vi "Oversampler.vi"(9 "Samplerate":dbl format="%#_13g", 10 "Array in":dbl[](array[numeric]), 11 "Oversampling":i32=15) -> (3 "Array out":dbl[](array[numeric]))   [LabVIEW 2016]
panel:
  out "Waveform Graph 2":dbl[](graph)
  out "Waveform Graph":dbl[](graph)
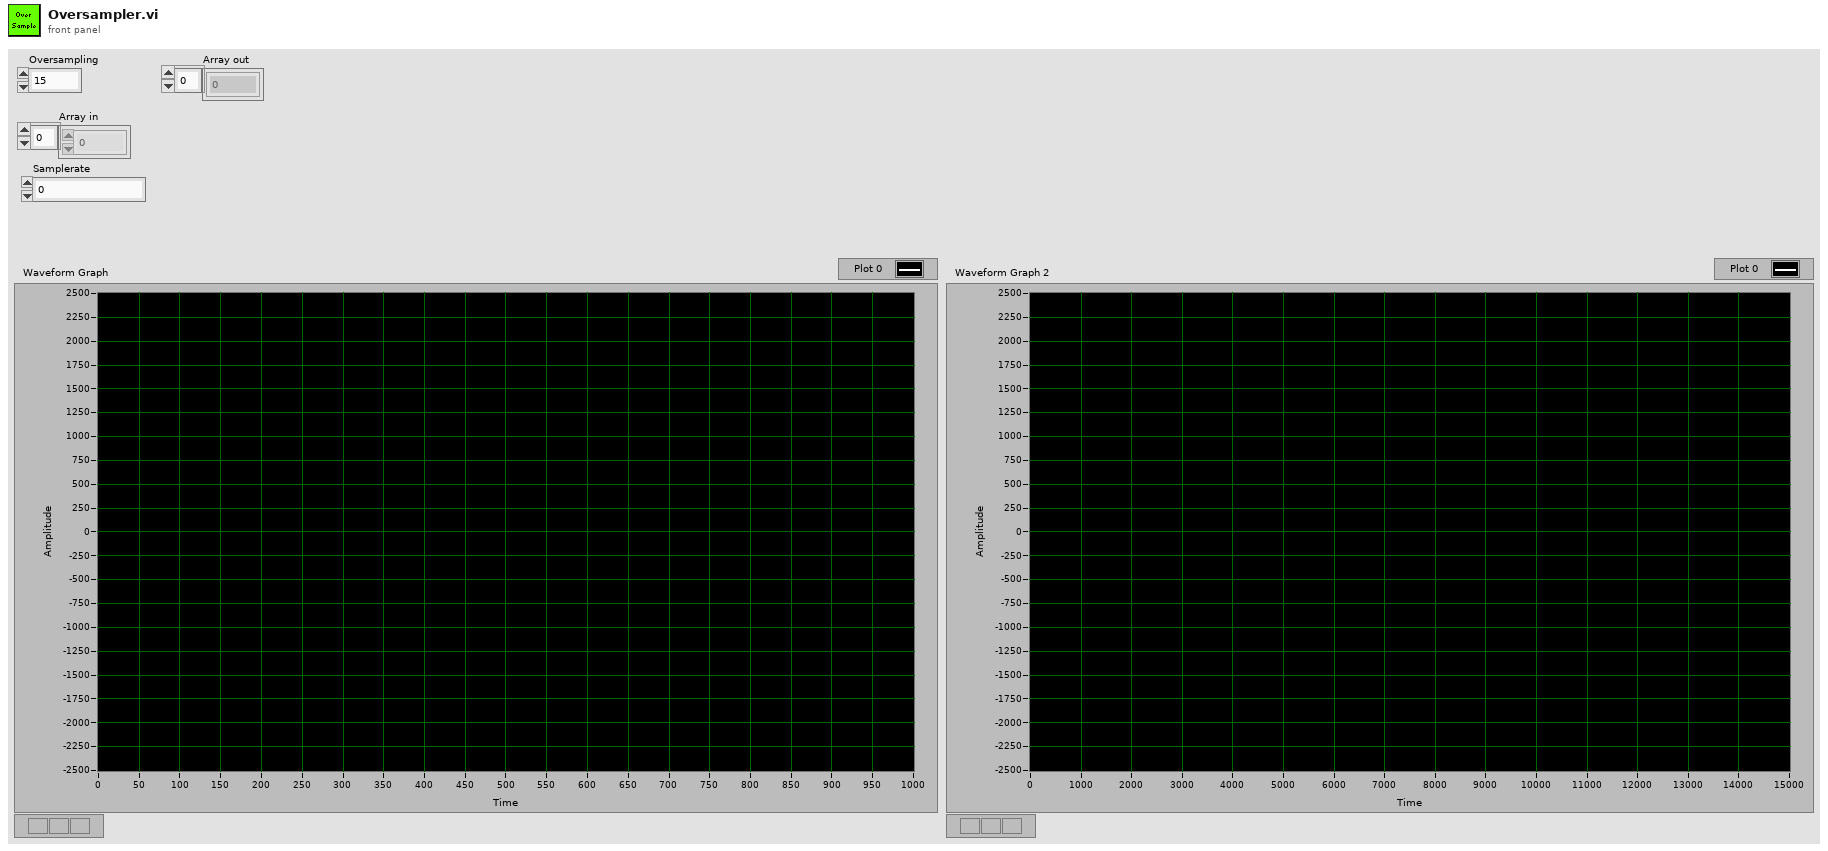
[diagram p1: front panel]
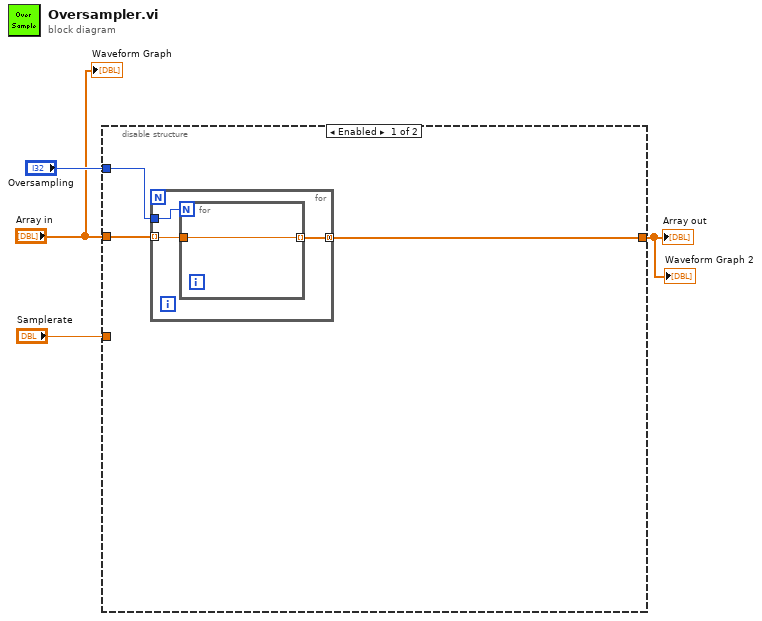
[diagram p0: block diagram]
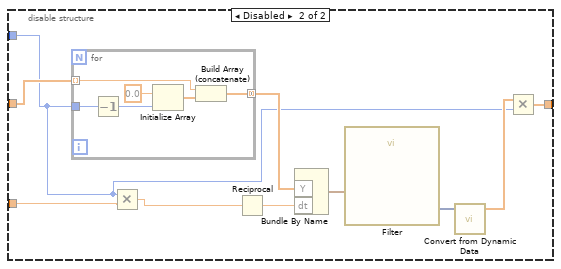
[diagram p2: hidden frame]
diagram:
  n1 = disable-structure shown="Enabled" {
    disable-tunnel: [w7 w12] -> w1
    disable-tunnel: "Oversampling" -> [w6 w13]
    disable-tunnel: "Array in" -> [w5 w21]
    disable-tunnel: "Samplerate" -> [_ w20]
    frame Enabled {
      n2 = for {
        tunnel: w5 -> [w9] mode=indexing
        tunnel: w6 -> [w10]
        tunnel: [w8] -> w7 mode=concatenating
        n3 = for {
          N: w10 -> [_]
          tunnel: w9 -> [w11]
          tunnel: [w11] -> w8 mode=indexing
        }
      }
    }
    frame Disabled {
      n4 = for {
        tunnel: w21 -> [w26] mode=indexing
        tunnel: w13 -> [w24]
        tunnel: [w22] -> w19 mode=concatenating
        n5 = Decrement(x=w24) -> (x-1=w23:i32)
        n6 = Initialize Array(0.0 ("element"), w23) -> (w25:dbl[])
        n7 = Build Array (concatenate)(w26, w25) -> (w22:dbl[])
      }
      n8 = Multiply(x=w13, y=w20) -> (x*y=w18:dbl)
      n9 = Reciprocal(x=w18) -> (1/x=w17:dbl)
      n10 = Bundle By Name("Y"=w19, "dt"=w17) -> (w16:waveform(dbl))  [unwired: 1 in]
      n11 = call "Filter"("Signal"=w16) -> ("Filtered Signal"=w15:dynamicdata)  [unwired: 9 in, 1 out]
      n12 = call "Convert from Dynamic Data"("Dynamic Data Type"=w15) -> ("Array"=w14:dbl[])  [unwired: 3 in]
      n13 = Multiply(x=w14, y=w13) -> (x*y=w12:dbl[])
    }
  }
  "Array out" <- w1
  "Waveform Graph 2" <- w1
  "Waveform Graph" <- "Array in"
